vi "fpga_LP2 Process (M Class_50Hz).vi"(0 "re":fxp<+/-,32,5> format="%.29g", 1 "reset":bool, 2 "Memory In":refnum<k21>="coefROM", 5 "im":fxp<+/-,32,5> format="%.29g", 7 "#Ch":fxp<+,5,5>=16.0, 9 "input valid":bool, 12 "ready for output":bool) -> (4 "re filtered":fxp<+/-,32,6> format="%.28g", 6 "im filtered":fxp<+/-,32,6> format="%.28g", 10 "output valid":bool, 14 "ready for input":bool, 15 "error":i32)   [LabVIEW 2013, in "NI_EP_PMU_FPGA.lvlib"]
uses:
  <vilib>/addons/Electrical Power/PMU/NI_EP_PMU_FPGA.lvlib
  <vilib>/rvi/FXPMathLib/basic elements/FxpDiscreteDelay/XNode/nifxpmath_DiscreteDelay.xnode
  <vilib>/addons/Electrical Power/PQ/Resampling/NI_EP_Resample_FPGA.lvlib
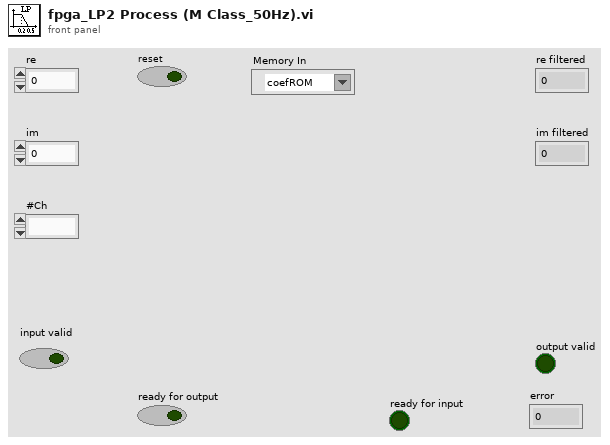
[diagram p1: front panel]
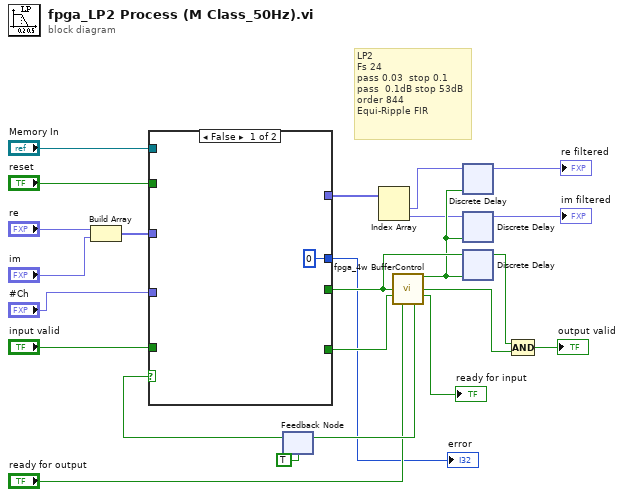
[diagram p0: block diagram]
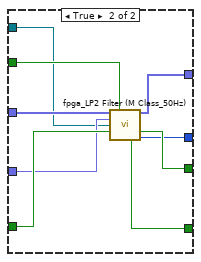
[diagram p2: hidden frame]
diagram:
  # "LP2\nFs 24\npass 0.03  stop 0.1\npass  0.1dB stop 53dB\norder 844\nEqui-Ripple FIR"
  n1 = Build Array("re", "im") -> (w6:fxp<+/-,32,5>[])
  n2 = feedback #1(TRUE ("logic enable")) -> (w19:bool)
  n3 = case shown="False" w19 {
    tunnel: "input valid" -> [_ w33]
    tunnel: "reset" -> [_ w30]
    tunnel: [_ w32] -> w13
    tunnel: [_ w28] -> w22
    tunnel: [_ w31] -> w5
    tunnel: w6 -> [_ w34]
    tunnel: "#Ch" -> [_ w29]
    tunnel: "Memory In" -> [_ w27]
    tunnel: [0 ("error") w26] -> w1
    frame False {
    }
    frame True {
      n4 = call <vilib>:"fpga_LP2 Filter (M Class_50Hz).vi"("input data"=w34, "reset"=w30, "#Ch"=w29, "Memory In"=w27, "input valid"=w33) -> ("output data"=w31:fxp<+/-,32,6>[], "output valid"=w32:bool, "ready for input"=w28:bool, "error"=w26:i32)  [unwired: 7 in]
    }
  }
  "error" <- w1
  n5 = Index Array(array=w5) -> (element #1=w4:fxp<+/-,32,6>, element #2=w3:fxp<+/-,32,6>)  [unwired: 2 in]
  n6 = call <vilib>:"fpga_4w BufferControl.vi"("DR"=w13, "RFI"=w22, "RFO"="ready for output") -> ("buff enable"=w10:bool, "output valid"=w21:bool, "ready for input"=→"ready for input":bool, "logic enable"=w20:bool)  [unwired: 9 in]
  n7 = feedback-in #1(w20) -> ()
  n8 = xnode ("Discrete Delay")("D"=w4, "enable"=w10) -> ("Q"=→"re filtered":fxp<+/-,32,6>)
  n9 = xnode ("Discrete Delay")("D"=w3, "enable"=w10) -> ("Q"=→"im filtered":fxp<+/-,32,6>)
  n10 = xnode ("Discrete Delay")("D"=w13, "enable"=w10) -> ("Q"=w12:bool)
  n11 = Compound Arithmetic op=AND(w12, w21) -> (→"output valid":bool)
